vi "UE fgv.vi"(7 "Set?":bool, 8 "error in (no error)":errorcluster) -> (0 "error out":errorcluster, 2 "UEs":T1, 3 "Event Registration Refnum":refnum<event-registration>)   [LabVIEW 2016]
uses:
  Controls/UEs.ctl
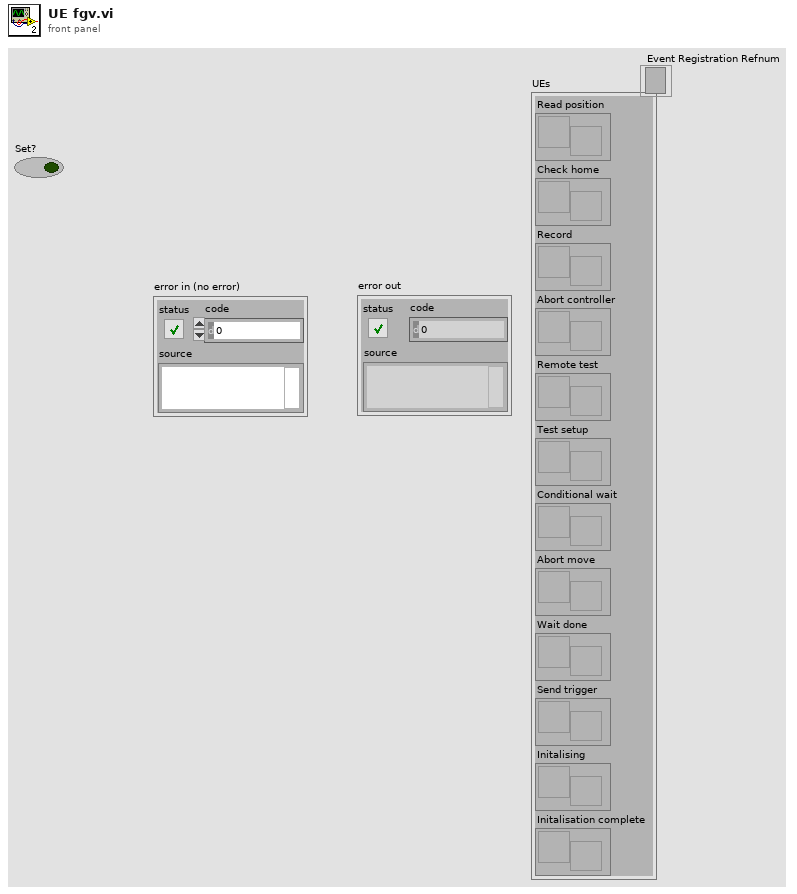
[diagram p1: front panel]
types:
  T1 = typedef "UEs.ctl" = cluster{"Read position":refnum<user-event>, "Check home":refnum<user-event>, "Record":refnum<user-event>, "Abort controller":refnum<user-event>, "Remote test":refnum<user-event>, "Test setup":refnum<user-event>, "Conditional wait":refnum<user-event>, "Abort move":refnum<user-event>, "Wait done":refnum<user-event>, "Send trigger":refnum<user-event>, "Initalising":refnum<user-event>, "Initalisation complete":refnum<user-event>}
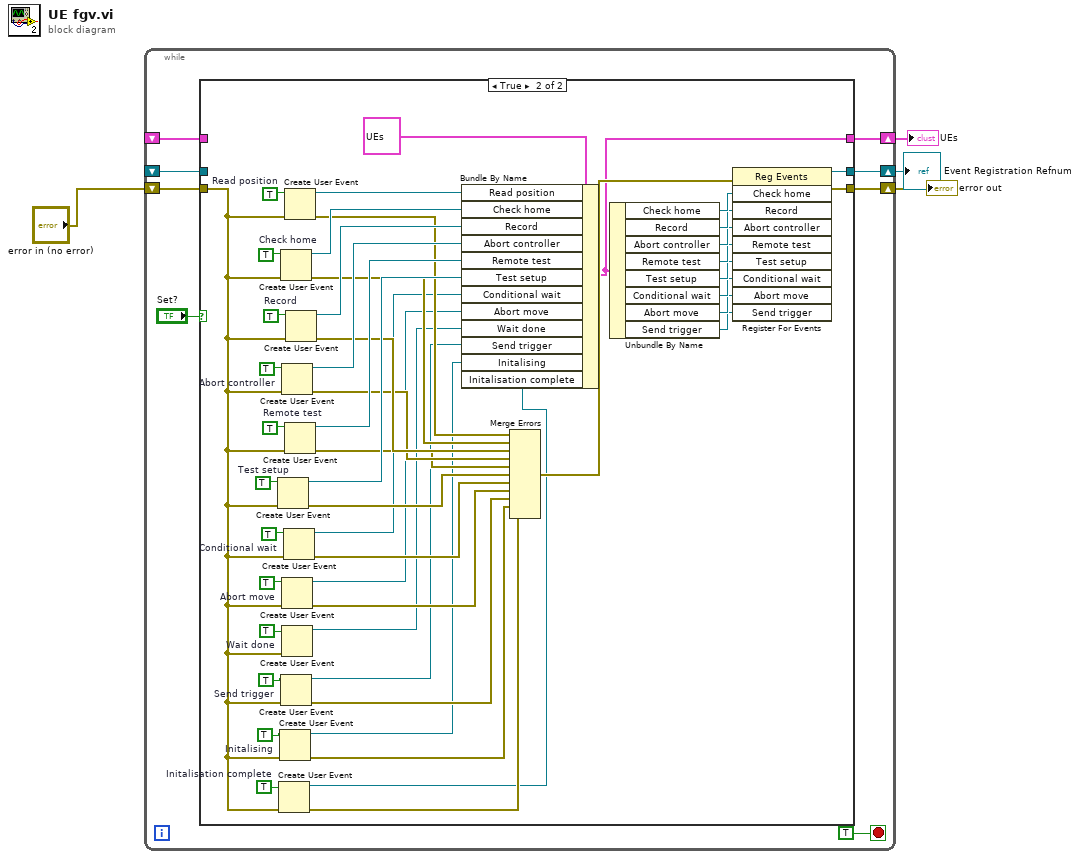
[diagram p0: block diagram]
diagram:
  n1 = while {
    shift-right: [w10] -> w3
    shift-left: "error in (no error)" -> [w11]
    shift-right: [w12] -> w1
    shift-left: _ -> [w5]
    shift-right: [w9] -> w2
    shift-left: _ -> [w6]
    stop <- TRUE stop-if-true
    n2 = case shown="True" "Set?" {
      tunnel: [w14 w46] -> w12
      tunnel: w11 -> [w13 w19]
      tunnel: [w13 w45] -> w10
      tunnel: [w15 w37] -> w9
      tunnel: w6 -> [w15 _]
      tunnel: w5 -> [w14 _]
      frame False {
      }
      frame True {
        w16 = TRUE  # Initalisation complete
        w22 = TRUE  # Initalising
        w26 = TRUE  # Send trigger
        w28 = TRUE  # Wait done
        w32 = TRUE  # Abort move
        w36 = TRUE  # Conditional wait
        w59 = TRUE  # Test setup
        w60 = TRUE  # Remote test
        w61 = TRUE  # Abort controller
        w62 = TRUE  # Check home
        w63 = TRUE  # Record
        w64 = TRUE  # Read position
        n3 = Create User Event(user event datatype=w59, error in=w19) -> (user event=w53:refnum<user-event>, error out=w39:errorcluster)
        n4 = Create User Event(user event datatype=w16, error in=w19) -> (user event=w17:refnum<user-event>, error out=w18:errorcluster)
        n5 = Create User Event(user event datatype=w22, error in=w19) -> (user event=w20:refnum<user-event>, error out=w21:errorcluster)
        n6 = Create User Event(user event datatype=w62, error in=w19) -> (user event=w57:refnum<user-event>, error out=w43:errorcluster)
        n7 = Create User Event(user event datatype=w26, error in=w19) -> (user event=w25:refnum<user-event>, error out=w24:errorcluster)
        n8 = Create User Event(user event datatype=w61, error in=w19) -> (user event=w55:refnum<user-event>, error out=w41:errorcluster)
        n9 = Create User Event(user event datatype=w32, error in=w19) -> (user event=w31:refnum<user-event>, error out=w30:errorcluster)
        n10 = Create User Event(user event datatype=w28, error in=w19) -> (user event=w27:refnum<user-event>)  [unwired: 1 out]
        n11 = Create User Event(user event datatype=w36, error in=w19) -> (user event=w34:refnum<user-event>, error out=w35:errorcluster)
        n12 = Create User Event(user event datatype=w64, error in=w19) -> (user event=w58:refnum<user-event>, error out=w44:errorcluster)
        n13 = Create User Event(user event datatype=w60, error in=w19) -> (user event=w54:refnum<user-event>, error out=w40:errorcluster)
        n14 = Create User Event(user event datatype=w63, error in=w19) -> (user event=w56:refnum<user-event>, error out=w42:errorcluster)
        n15 = Bundle By Name(cluster=T1 {"Read position"=refnum, "Check home"=refnum, "Record"=refnum, "Abort controller"=refnum, "Remote test"=refnum, "Test setup"=refnum, "Conditional wait"=refnum, "Abort move"=refnum, "Wait done"=refnum, "Send trigger"=refnum, "Initalising"=refnum, "Initalisation complete"=refnum}, "Read position"=w58, "Check home"=w57, "Record"=w56, "Abort controller"=w55, "Remote test"=w54, "Test setup"=w53, "Conditional wait"=w34, "Abort move"=w31, "Wait done"=w27, "Send trigger"=w25, "Initalising"=w20, "Initalisation complete"=w17) -> (w37:T1)
        n16 = Merge Errors(w44, w43, w42, w41, w40, w39, w35, w30, w24, w21, w18) -> (w38:errorcluster)
        n17 = Unbundle By Name(w37) -> ("Check home"=w51:refnum<user-event>, "Record"=w50:refnum<user-event>, "Abort controller"=w49:refnum<user-event>, "Remote test"=w48:refnum<user-event>, "Test setup"=w47:refnum<user-event>, "Conditional wait"=w33:refnum<user-event>, "Abort move"=w29:refnum<user-event>, "Send trigger"=w23:refnum<user-event>)
        n18 = register-events(error in=w38, w51, w50, w49, w48, w47, w33, w29, w23) -> (reference out=w46:refnum<event-registration>, error out=w45:errorcluster)  [unwired: 1 in]
      }
    }
  }
  "error out" <- w3
  "UEs" <- w2
  "Event Registration Refnum" <- w1
